vi "trio_home_status.vi"(8 "error in":errorcluster, 11 "reference in":refnum<k7>) -> (0 "Error out":errorcluster, 2 "Status":T1, 3 "reference out":refnum<k7>)   [LabVIEW 2017]
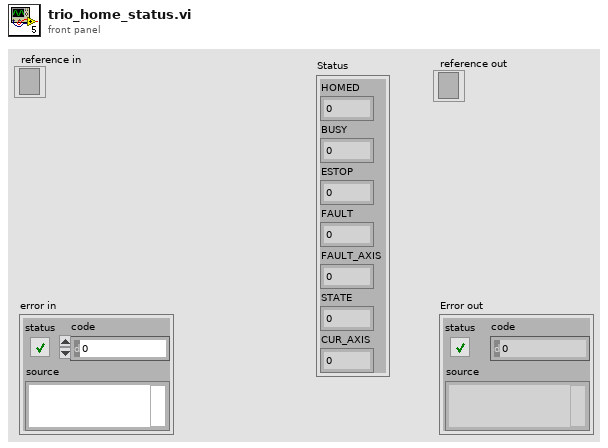
[diagram p1: front panel]
types:
  T1 = cluster{"HOMED":dbl, "BUSY":dbl, "ESTOP":dbl, "FAULT":dbl, "FAULT_AXIS":dbl, "STATE":dbl, "CUR_AXIS":dbl}
  T2 = cluster{"[0]":dbl, "[1]":dbl, "[2]":dbl, "[3]":dbl, "[4]":dbl, "[5]":dbl, "[6]":dbl}
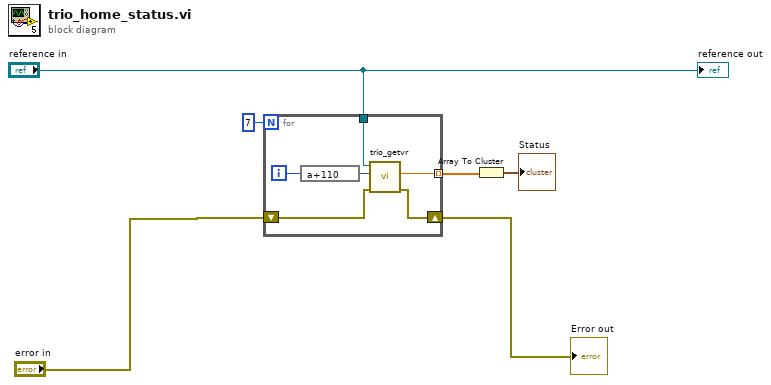
[diagram p0: block diagram]
diagram:
  n1 = for {
    N: 7 -> [_]
    shift-right: [w9] -> w1
    shift-left: "error in" -> [w10]
    tunnel: "reference in" -> [w8]
    tunnel: [w7] -> w3 mode=indexing
    i -> [w11]
    n2 = expression code="a+110"(w11) -> (w12:i32)
    n3 = call "trio_getvr.vi"("error in (no error)"=w10, "Vr #"=w12, "reference in"=w8) -> ("error out"=w9:errorcluster, "Value"=w7:dbl)  [unwired: 5 in, 2 out]
  }
  "Error out" <- w1
  n4 = Array To Cluster(array=w3) -> (cluster=→"Status":T2)
  "reference out" <- "reference in"
